vi "Differential Steering Demonstrator.vi"() -> ()   [LabVIEW 2011]
panel:
  out "Right":dbl
  out "Left":dbl
  in  "Base":dbl=0.85 step=0.1
  in  "Steer":dbl(knob) scale=-1.2..1.2
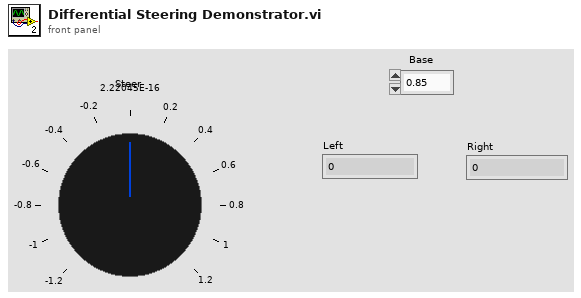
[diagram p1: front panel]
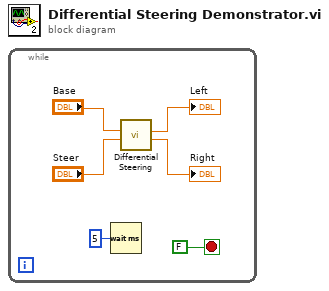
[diagram p0: block diagram]
diagram:
  n1 = while {
    stop <- FALSE stop-if-true
    n2 = Wait (ms)(milliseconds to wait=u32 5) -> ()  [unwired: 1 out]
    n3 = call "Differential Steering.vi"("Steer"="Steer", "Base"="Base") -> ("Right"=→"Right":dbl, "Left"=→"Left":dbl)  [unwired: 4 in]
  }
